vi "Generate DGML header.vi"(11 "Create Unowned Container?":bool) -> (3 "String":string)   [LabVIEW 2018, in "DGML creation.lvlib"]
uses:
  DGML creation.lvlib
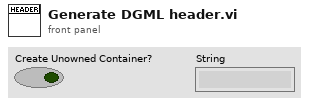
[diagram p1: front panel]
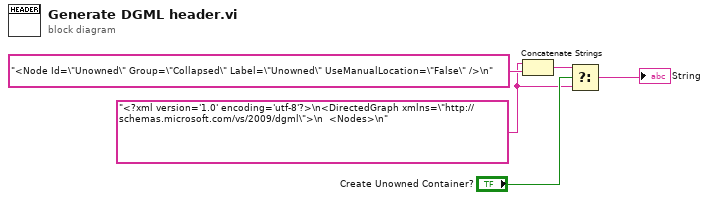
[diagram p0: block diagram]
diagram:
  w2 = "<?xml version='1.0' encoding='utf-8'?>\n<DirectedGraph xmlns=\"http://schemas.microsoft.com/vs/2009/dgml\">\n  <Nodes>\n"
  n1 = Concatenate Strings(w2, "<Node Id=\"Unowned\" Group=\"Collapsed\" Label=\"Unowned\" UseManualLocation=\"False\" />\n" ("string")) -> (w1:string)
  n2 = Select(t=w1, s="Create Unowned Container?", f=w2) -> (s? t:f=→"String":string)
